vi "simpleOrderAnalysis.vi"() -> ()   [LabVIEW 2019]
uses:
  <vilib>/addons/Sound and Vibration/Order Analysis/Utility/SoundVib_OAUtility.lvlib
  <vilib>/addons/Sound and Vibration/Order Analysis/Tach Process/SoundVib_TachProcess.lvlib
  <vilib>/addons/Sound and Vibration/Order Analysis/Resample Order Tracking/SoundVib_OrderTracking.lvlib
  <vilib>/myRIO/Common/Instrument Driver Framework/myRIO v1.0/DIO/typedefs/DIO Channels Enum.ctl
  <vilib>/myRIO/Common/Instrument Driver Framework/myRIO v1.0/DIO/typedefs/DIO Channels List.ctl
  <vilib>/myRIO/Common/Instrument Driver Framework/Utilities/typedefs/Generic FPGA Reference.ctl
  <vilib>/myRIO/Common/Instrument Driver Framework/Utilities/typedefs/myRIO v1.0 Reference.ctl
  <vilib>/myRIO/Common/Instrument Driver Framework/Utilities/typedefs/Hardware Version Enum.ctl
  <vilib>/myRIO/Common/Instrument Driver Framework/Utilities/typedefs/myRIO Generic Hardware Reference.ctl
  <vilib>/myRIO/Instrument Drivers/Onboard IO/DIO/typedefs/DIO Reference.ctl
  <vilib>/myRIO/Instrument Drivers/Onboard IO/DIO/DIO.lvlib
  <vilib>/myRIO/Instrument Drivers/Onboard IO/DIO/vis/myRIO DIO Open.xnode
  <vilib>/myRIO/Common/Instrument Driver Framework/myRIO v1.0/DIO/vis/myRIO v1.1 Open DIO.vi
  <vilib>/userdefined/High Color/nirio_resource_hc.ctl
  <vilib>/platform/TimedLoop/XDataNode/XDataNode.xnode
  <vilib>/Platform/TimedLoop/XDataNode/nitl_modes.ctl
  <vilib>/Platform/TimedLoop/XDataNode/XDNodeRunTimeDep.lvlib
  <vilib>/Platform/TimedLoop/XDataNode/wakeup.ctl
  <vilib>/Platform/TimedLoop/XDataNode/timing_clust.ctl
  <vilib>/addons/Sound and Vibration/Order Analysis/Utility/OAT Output Triggered Even Angle Signal (1 Channel).vi
  <vilib>/addons/Sound and Vibration/Order Analysis/Tach Process/OAT Analog Tacho Process (1 Tacho).vi
  <vilib>/addons/Sound and Vibration/Order Analysis/Resample Order Tracking/OAT Convert to Even Angle Signal (1 Channel).vi
  <vilib>/addons/Sound and Vibration/Order Analysis/Resample Order Tracking/OAT Order Power Spectrum (1 Channel).vi
  <vilib>/addons/_NISVFA/_Spectrum Processing/SVFA Power in Band (1 Ch).vi
panel:
  in  "stop":bool
  in  "order resolution":dbl=0.1 min=0.0 format="%.3f"
  out "powers in band":dbl[](array[numeric]) format="%.2f"
  in  "order range":cluster{"start":dbl, "stop":dbl}={"start"=-1.0, "stop"=-1.0} {"stop" format="%.2f"; "start" format="%.2f"}
  out "actual max order":dbl
  in  "window type":u32(ring)=1 items=["None"=0, "Hanning"=1, "Hamming"=2, "Blackman-Harris"=3, "Exact Blackman"=4, "Blackman"=5, "Flat Top"=6, "4 Term B-Harris"=7, "7 Term B-Harris"=8, "Low Sidelobe"=9, "Gaussian"=62]
  in  "max order to analyze":i32=32
  out "Speed profile":cluster{"time [s]":dbl[], "speed [RPM]":dbl[]}(graph)
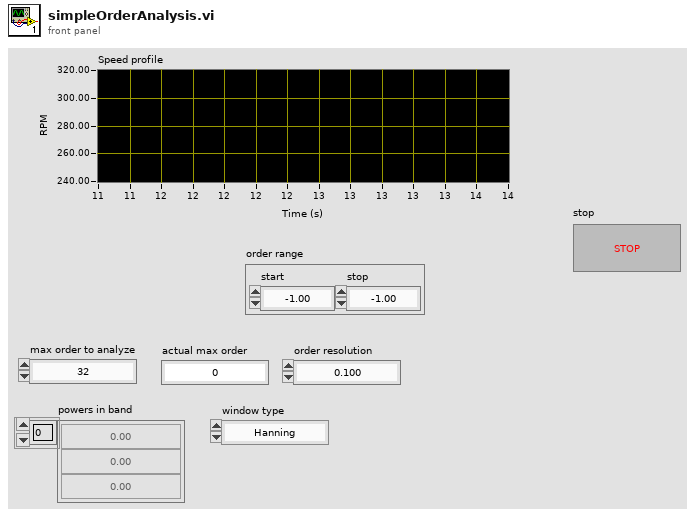
[diagram p1: front panel]
types:
  T1 = cluster{"averaging mode":enum16{"No averaging", "Vector averaging", "RMS averaging", "Peak hold"}, "weighting mode":enum16{"Linear", "Exponential"}, "number of averages":u32, "linear mode":enum16{"One shot", "Auto restart"}}
  T2 = typedef "DIO.lvlib/DIO Reference.ctl" = cluster{"myRIO Reference":T3, "DIO Channels List":T7}
  T3 = typedef "myRIO Generic Hardware Reference.ctl" = cluster{"myRIO Model":T4, "myRIO Hardware Reference":T5}
  T4 = typedef "Hardware Version Enum.ctl" = enum16{"Unknown", "myRIO-1900", "myRIO-1950", "roboRIO", "NI ELVIS RIO CM", "ELVIS III"}
  T5 = typedef "myRIO v1.0 Reference.ctl" = cluster{"Generic FPGA Reference":T6, "Allow multiple opens":bool}
  T6 = typedef "Generic FPGA Reference.ctl" = refnum<k20>
  T7 = typedef "DIO Channels List.ctl" = T8[]
  T8 = typedef "DIO Channels Enum.ctl" = enum16{"Not Connected", "C/DIO0", "C/DIO1", "C/DIO2", "C/DIO3", "C/DIO4", "C/DIO5", "C/DIO6", "C/DIO7", "A/DIO0", "A/DIO1", "A/DIO2", "A/DIO3", "A/DIO4", "A/DIO5", "A/DIO6", "A/DIO7", "A/DIO8", "A/DIO9", "A/DIO10", "A/DIO11", "A/DIO12", "A/DIO13", "A/DIO14", "A/DIO15", "A/DIO16", "A/DIO17", "A/DIO18", "A/DIO19", "B/DIO0", "B/DIO1", "B/DIO2", "B/DIO3", "B/DIO4", "B/DIO5", "B/DIO6", "B/DIO7", "B/DIO8", "B/DIO9", "B/DIO10", "B/DIO11", "B/DIO12", "B/DIO13", "B/DIO14", "B/DIO15", "B/DIO16", "B/DIO17", "B/DIO18", "B/DIO19", "LED0", "LED1", "LED2", "LED3", "Button0", "DIO/DIO0", "DIO/DIO1", "DIO/DIO2", "DIO/DIO3", "DIO/DIO4", "DIO/DIO5", "DIO/DIO6", "DIO/DIO7", "DIO/DIO8", "DIO/DIO9", "SPI/CS0", "SPI/CS1", "SPI/CS2", "SPI/CS3", "LED RADIO (Green)", "LED RADIO (Red)", "LED COMM (Green)", "LED COMM (Red)", "LED MODE (Green)", "LED MODE (Red)"}
  T9 = typedef "XDNodeRunTimeDep.lvlib/timing_clust.ctl" = cluster{"Expected End [f-1]":u64, "Actual End [f-1]":u64, "Finished Late? [f-1]":bool, "Expected End [i-1]":u64, "Actual End [i-1]":u64, "Finished Late? [i-1]":bool, "Expected Start [i]":u64, "Actual Start [i]":u64, "Expected Start [f]":u64, "Actual Start [f]":u64, "Source Name":string, "Structure Name":string, "Period":i64, "Deadline":i64, "Offset":i64, "Start":i64, "Priority":i32, "Timeout":i32, "Mode":T10, "Wakeup Reason":T11, "Error":errorcluster, "Source Type":string, "Secondary Source Type":string, "Global End Time":u64, "Global Start Time":u64, "Frame Duration":u64, "Iteration Duration":u64, "Assigned CPU":i32, "I/O Scan Engine Mode":u32}
  T10 = typedef "XDNodeRunTimeDep.lvlib/nitl_modes.ctl" = enum32{"No Change", "Process missed periods, maintain original phase", "Discard missed periods, maintain original phase", "Process missed periods, ignore original phase", "Discard missed periods, ignore original phase"}
  T11 = typedef "XDNodeRunTimeDep.lvlib/wakeup.ctl" = enum32{"Normal", "Aborted", "Asynchronous wakeup", "Timing source error", "Timed loop error", "Timeout"}
  T12 = typedef "SoundVib_TachProcess.lvlib/speed profile.ctl" = cluster{"time [s]":dbl[], "speed [RPM]":dbl[]}
  T13 = typedef "svc_Resampled Channel Info.ctl" = cluster{"channel name":string, "description":string, " channel info":T14}
  T14 = typedef "svc_Channel Info.ctl" = cluster{"sensor sensitivity":dbl, "engineering units":T15, "dB reference":dbl, "custom label":string, "weighting filter":T16, "pregain":dbl}
  T15 = typedef "svc_Engineering Units Text Ring.ctl" = u16
  T16 = typedef "svc_Weighting Filter Text Ring.ctl" = u16
  T17 = cluster{"order 0":dbl, "delta order":dbl, "magnitude":dbl[]}
  T18 = typedef "svc_Spectrum Info.ctl" = cluster{"channel name":string, "description":string, "x-axis units":T19, "spectral info":cluster{"spectrum type":T20, "linear/dB":enum16{"linear", "dB"}, "window":u16, "window size":i32, "FFT size":i32}, "engineering units":T15, "custom label":string, "dB reference [EU]":dbl, "peak units":enum16{"rms", "peak", "peak-peak"}, "weighting filter":T16, "spectral density?":bool, "unit label":string, "spectrum skewed?":bool, "complimentary spectrum units":T21}
  T19 = typedef "svc_X-Axis Units.ctl" = u16
  T20 = typedef "svc_Spectrum Type.ctl" = enum16{"FFT Spectrum [complex]", "Amplitude [Magnitude]", "Power [Magnitude^2]", "Cross Spectrum [complex]", "Frequency Response [Complex]"}
  T21 = typedef "svc_Complimentary Spectrum Units.ctl" = enum16{"none", "radians", "degrees", "cycles", "imaginary"}
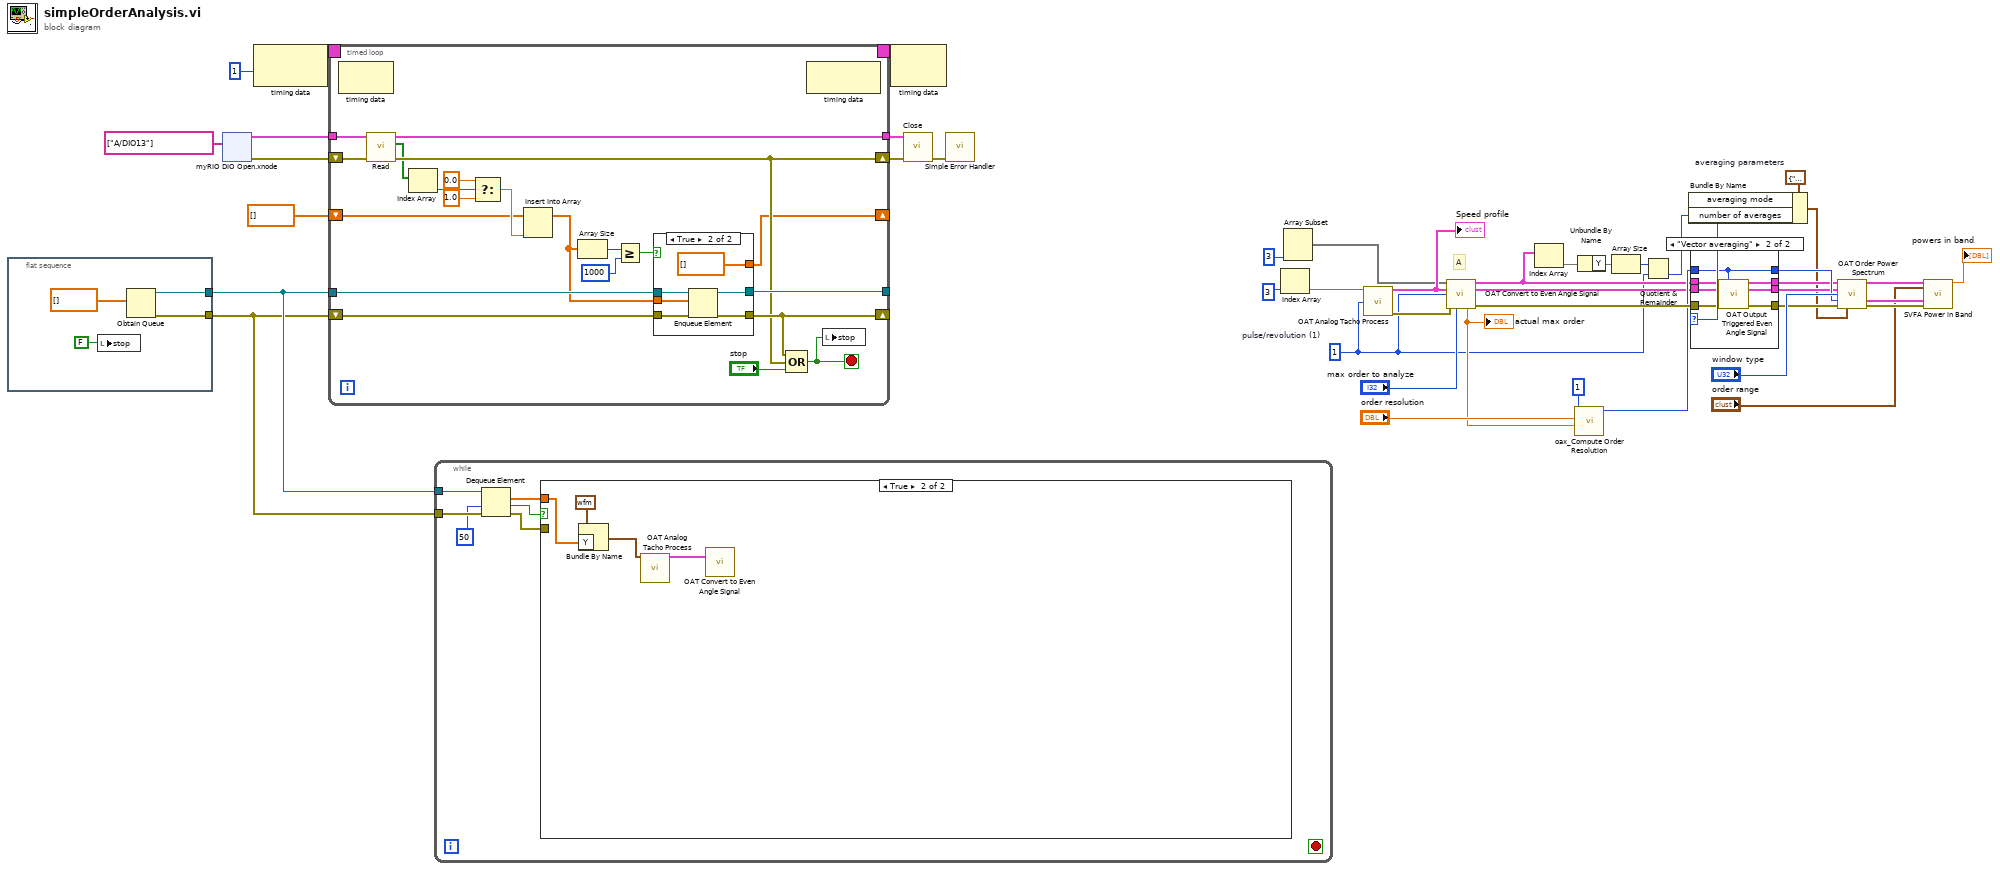
[diagram p0: block diagram]
diagram:
  w19 = 1  # pulse/revolution (1)
  w31 = T1 {"averaging mode"=enum."RMS averaging", "weighting mode"=enum."Linear", "number of averages"=10, "linear mode"=enum."One shot"}  # averaging parameters
  # "A"
  n1 = flat-sequence {
    tunnel: [w53] -> w3
    tunnel: [w52] -> w2
    frame #0 {
      n2 = local write "stop"(FALSE ("stop")) -> ()
      n3 = Obtain Queue(element data type=dbl[] []) -> (queue out=w53:refnum<queue>, error out=w52:errorcluster)  [unwired: 4 in, 1 out]
    }
  }
  n4 = xnode "myRIO DIO Open.xnode"("Channel Names"=tag[] ["A/DIO13"]) -> ("error out"=w11:errorcluster, "DIO Ref Out"=w10:T2)  [unwired: 2 in]
  n5 = node-c288(i64 1 ("Period")) -> (w9:T9)
  n6 = timed-loop {
    tunnel: w10 -> [w74]
    shift-right: [w62] -> w6
    shift-left: w11 -> [w73]
    timing: w9 -> [_]
    timing-out: [_] -> w8
    tunnel: [w72] -> w5
    shift-right: [w54] -> _
    shift-left: dbl[] [] -> [w55]
    tunnel: w3 -> [w69]
    tunnel: [w65] -> _
    shift-right: [w63] -> _
    shift-left: w2 -> [w68]
    stop <- w61 stop-if-true
    n7 = node-c288() -> ()  [unwired: 1 in, 1 out]
    n8 = call <vilib>:"Read.vi"("error in (no error)"=w73, "DIO Ref In"=w74) -> ("error out"=w62:errorcluster, "Values"=w60:bool[], "DIO Ref Out"=w72:T2)  [unwired: 7 in]
    n9 = Index Array(array=w60) -> (element=w59:bool)  [unwired: 1 in]
    n10 = Select(t=0.0, s=w59, f=1.0) -> (s? t:f=w56:dbl)
    n11 = Insert Into Array(array=w55, new element=w56) -> (w66:dbl[])  [unwired: 1 in]
    n12 = Array Size(array=w66) -> (size(s)=w71:i32)
    n13 = Greater Or Equal?(x=w71, y=1000) -> (x >= y?=w67:bool)
    n14 = case shown="True" w67 {
      tunnel: w69 -> [w77 w83]
      tunnel: w68 -> [w76 w82]
      tunnel: w66 -> [w75 w79]
      tunnel: [w77 w81] -> w65
      tunnel: [w76 w80] -> w63
      tunnel: [w75 dbl[] []] -> w54
      frame False {
      }
      frame True {
        n15 = Enqueue Element(queue=w83, element=w79, error in (no error)=w82) -> (queue out=w81:refnum<queue>, error out=w80:errorcluster)  [unwired: 1 in, 1 out]
      }
    }
    n16 = Compound Arithmetic op=OR(w63, w62, "stop") -> (w61:bool)
    n17 = node-c288() -> ()  [unwired: 1 in, 1 out]
    n18 = local write "stop"(w61) -> ()
  }
  n19 = while {
    tunnel: w3 -> [w91]
    tunnel: w2 -> [w90]
    stop <- _ stop-if-true
    n20 = Dequeue Element(queue=w91, timeout in ms (-1)=50, error in (no error)=w90) -> (element=w87:dbl[], timed out?=w88:bool, error out=w86:errorcluster)  [unwired: 1 out]
    n21 = case shown="True" w88 {
      tunnel: w87 -> [_ w94]
      tunnel: w86 -> [_ _]
      frame False {
      }
      frame True {
        n22 = Bundle By Name(cluster=waveform(dbl) {"t0"=timestamp(0 s since 1904-01-01), "dt"=0.0, "Y"=[]} ("analog tacho signal"), "Y"=w94) -> (w93:waveform(dbl))
        n23 = call-poly <vilib>:"OAT Analog Tacho Process.vi"("analog tacho signal"=w93) -> ("speed profile"=w92:T12)  [unwired: 10 in, 4 out]
        n24 = call-poly <vilib>:"OAT Convert to Even Angle Signal.vi"("speed profile"=w92) -> ()  [unwired: 10 in, 5 out]
      }
    }
  }
  n25 = node-c288(w8) -> ()  [unwired: 1 out]
  n26 = call <vilib>:"Close.vi"("error in (no error)"=w6, "DIO Ref In"=w5) -> ("error out"=w4:errorcluster)  [unwired: 9 in]
  n27 = call <vilib>:"Simple Error Handler.vi"("error in (no error)"=w4) -> ()  [unwired: 4 in, 5 out]
  n28 = Index Array(index=3) -> (array=w21:waveform(dbl)[], element=w24)
  n29 = Array Subset(length=3) -> (array=w22:dbl[], w13:void[])  [unwired: 1 in]
  n30 = call-poly <vilib>:"OAT Analog Tacho Process.vi"("analog tacho signal"=w24, "pulse/revolution (1)"=w19) -> ("speed profile"=w49:T12, "error in (no error)"=w14:errorcluster, "error out"=w42:errorcluster)  [unwired: 8 in, 3 out]
  "Speed profile" <- w49
  n31 = call-poly <vilib>:"OAT Convert to Even Angle Signal.vi"("scaled signal [EU]"=w13, "speed profile"=w49, "pulse/revolution (1)"=w19, "error in (no error)"=w42, "max order (auto)"="max order to analyze") -> ("even-angle signal"=w30:cluster{"r0":dbl, "dr":dbl, "Y":dbl[]}, "even-angle channel info"=w36:T13, "actual max order"=w32:dbl, "error out"=w40:errorcluster)  [unwired: 6 in, 1 out]
  "actual max order" <- w32
  n32 = Index Array(array=w30) -> (element=w29)  [unwired: 1 in]
  n33 = call <vilib>:"oax_Compute Order Resolution.vi"("actual max order"=w32, "order resolution"="order resolution", "block size"=1) -> ("block size out"=w38:i32)  [unwired: 7 in, 1 out]
  n34 = Unbundle By Name(w29) -> ("Y"=w28)
  n35 = Array Size(array=w28) -> (size(s)=w27:i32)
  n36 = Quotient & Remainder(x=w27, y=w19) -> (floor(x/y)=w26:i32)  [unwired: 1 out]
  n37 = case shown="\"Vector averaging\"" w15 {
    tunnel: w40 -> [w98 w106]
    tunnel: [w98 w105] -> w39
    tunnel: w38 -> [w99 w104]
    tunnel: [w99 w104] -> w37
    tunnel: w30 -> [w96 w103]
    tunnel: w36 -> [w97 w102]
    tunnel: [w97 w100] -> w35
    tunnel: [w96 w101] -> w34
    frame "No averaging", Default {
    }
    frame "Vector averaging" {
      n38 = call-poly <vilib>:"OAT Output Triggered Even Angle Signal.vi"("even-angle signal"=w103, "block size"=w104, "even-angle channel info"=w102, "error in (no error)"=w106) -> ("triggered even-angle signal"=w101:cluster{"r0":dbl, "dr":dbl, "Y":dbl[]}, "even-angle channel info out"=w100:T13, "error out"=w105:errorcluster)  [unwired: 9 in]
    }
  }
  n39 = Bundle By Name(cluster=w31, "averaging mode"=w15, "number of averages"=w26) -> (w25:T1)
  n40 = call-poly <vilib>:"OAT Order Power Spectrum.vi"("even-angle signal"=w34, "even-angle channel info"=w35, "window"="window type", "block size"=w37, "error in (no error)"=w39, "averaging parameters"=w25) -> ("dB on? (T)"=w16:bool, "order power spectrum"=w17:T17, "spectrum info"=w46:T18, "error out"=w45:errorcluster)  [unwired: 2 in, 4 out]
  n41 = call-poly <vilib>:"SVFA Power in Band.vi"("spectrum"=w17, "range"="order range", "spectrum info"=w46, "error in (no error)"=w45) -> ("power in band"=→"powers in band":dbl, "error out"=w18:errorcluster)  [unwired: 13 in, 1 out]
